vi "ProcessingLoop.vi"(8 "error in (no error)":errorcluster, 11 "navX in":refnum<class "navX.lvclass">) -> (0 "error out":errorcluster, 3 "navX out":refnum<class "navX.lvclass">)   [LabVIEW 2015, in "navX Library v3.lvlib" / "navX.lvclass"]
uses:
  navX.lvclass
  navX.lvclass/navX.ctl
  navX - Base/navX - Base.lvclass
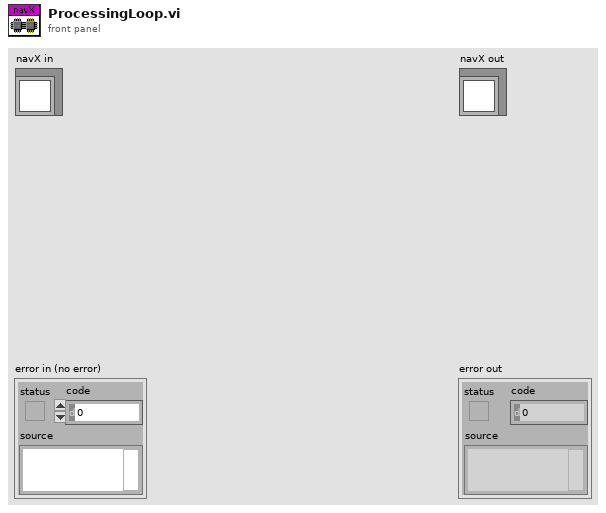
[diagram p1: front panel]
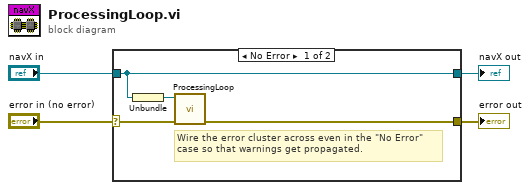
[diagram p0: block diagram]
diagram:
  n1 = case shown="No Error" "error in (no error)" {
    selector: "error in (no error)" -> [w6 w10]
    tunnel: [w7 w10] -> w3
    tunnel: [w8 w9] -> w1
    tunnel: "navX in" -> [w8 w9]
    frame No Error {
      # "Wire the error cluster across even in the \"No Error\"\ncase so that warnings get propagated."
      n2 = Unbundle(w8) -> (w5:refnum<class "navX - Base.lvclass">)
      n3 = call-dynamic "ProcessingLoop.vi"("error in (no error)"=w6, "navX - Base in"=w5) -> ("error out"=w7:errorcluster)  [unwired: 8 in, 1 out]
    }
    frame Error {
    }
  }
  "error out" <- w3
  "navX out" <- w1
